vi "Analyze (static).vi"(8 "error in (no error)":errorcluster, 10 "Image in":T1, 11 "Analyze Energy in":refnum<class "Analyze Energy.lvclass">) -> (0 "error out":errorcluster, 1 "Result":refnum<class "Analyze Results Energy.lvclass">, 2 "Image out":T1, 3 "Analyze Energy out":refnum<class "Analyze Energy.lvclass">)   [LabVIEW 2014, in "Analyze.lvlib" / "Analyze Energy.lvclass"]
uses:
  Analyze Energy.lvclass
  <vilib>/vision/Image Controls.llb/IMAQ Image.ctl
  Results and Overlays/Results Energy/Analyze Results Energy.lvclass
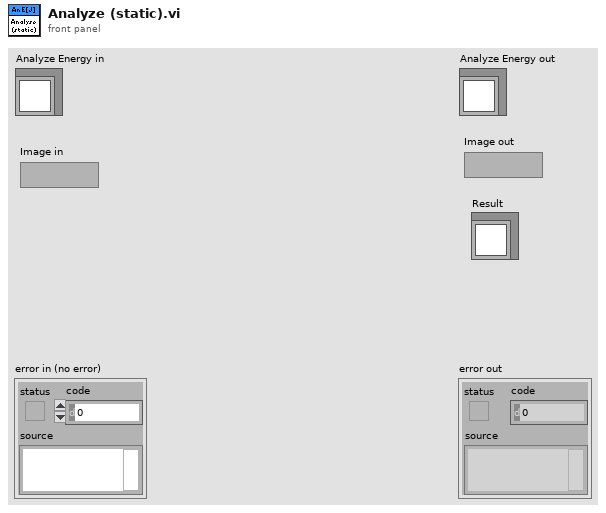
[diagram p1: front panel]
types:
  T1 = typedef "IMAQ Image.ctl" = refnum<image>
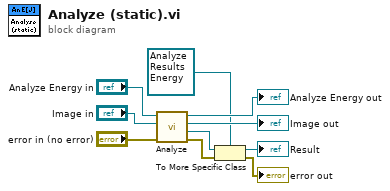
[diagram p0: block diagram]
diagram:
  n1 = call-dynamic "Analyze.vi"("error in (no error)"="error in (no error)", "Image in"="Image in", "Analyze Energy in"="Analyze Energy in") -> ("error out"=w5:errorcluster, "Result"=w2:refnum<class "Analyze Results Base.lvclass">, "Image out"=→"Image out":T1, "Analyze Energy out"=→"Analyze Energy out":refnum<class "Analyze Energy.lvclass">)  [unwired: 5 in]
  n2 = To More Specific Class(target class=refnum<class "Analyze Results Energy.lvclass"> refnum ("Analyze Results Energy.lvclass"), reference=w2, error in=w5) -> (specific class reference=→"Result":refnum<class "Analyze Results Energy.lvclass">, error out=→"error out":errorcluster)
